vi "WPI_InterruptOpen.vi"(8 "error in (no error)":errorcluster, 9 "Falling Edge":bool, 10 "Rising Edge":bool, 11 "Source":T1={"DevStatus"={"status"=FALSE, "code"=0, "source"=""}, "AnalogTriggerMode?"=FALSE, "DigitalMode"={"DIO Channel"=enum."Disabled"}, "AnalogTriggerMode"={"AnalogTriggerIndex"=enum."Trig 0", "OutputType"=enum."InWindow"}}) -> (0 "error out":errorcluster, 3 "InterruptRef":T5={"DevStatus"={"status"=FALSE, "code"=0, "source"=""}, "InterruptIndex"=enum."Invalid"})   [LabVIEW 2017]
doc: "Opens a reference to the interrupt you specify. You must open a reference before using any other VIs on this palette.\n\nThis software is licensed. Open the labview\\readme\\WPI Robotics Library Open Source License.txt file for more information."
uses:
  <vilib>/Rock Robotics/WPI/Interrupt/WPI_InterruptRef.ctl
  <vilib>/Rock Robotics/SystemInterfaces/Interrupt/FPGA_InterruptIndex.ctl
  <vilib>/Rock Robotics/SystemInterfaces/CounterEncoderSourceConvertion/FPGA_CounterEncoderSourceConvertionLVSourceType.ctl
  <vilib>/Rock Robotics/SystemInterfaces/DIO/FPGA_DIODigitalSourceChannel.ctl
  <vilib>/Rock Robotics/SystemInterfaces/AnalogTrigger/FPGA_AnalogTriggerIndex.ctl
  <vilib>/Rock Robotics/SystemInterfaces/AnalogTrigger/FPGA_AnalogTriggerOutType.ctl
  <vilib>/Rock Robotics/WPI/Interrupt/WPI_InterruptCacheOp.ctl
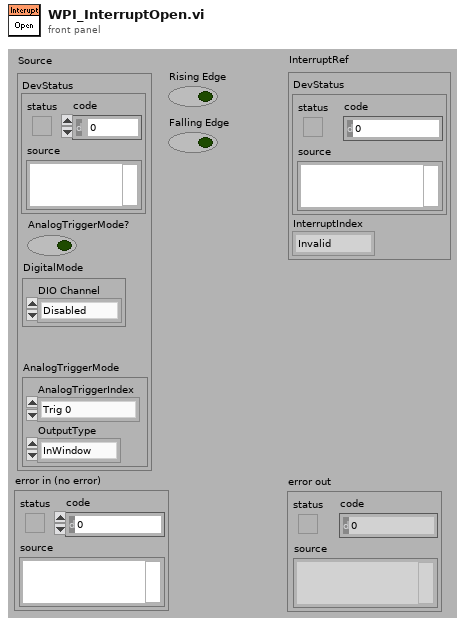
[diagram p1: front panel]
types:
  T1 = typedef "FPGA_CounterEncoderSourceConvertionLVSourceType.ctl" = cluster{"DevStatus":errorcluster, "AnalogTriggerMode?":bool, "DigitalMode":cluster{"DIO Channel":T2}, "AnalogTriggerMode":cluster{"AnalogTriggerIndex":T3, "OutputType":T4}}
  T2 = typedef "FPGA_DIODigitalSourceChannel.ctl" = enum8{"DIO 0", "DIO 1", "DIO 2", "DIO 3", "DIO 4", "DIO 5", "DIO 6", "DIO 7", "DIO 8", "DIO 9", "DIO MXP 0", "DIO MXP 1", "DIO MXP 2", "DIO MXP 3", "DIO MXP 4", "DIO MXP 5", "DIO MXP 6", "DIO MXP 7", "DIO MXP 8", "DIO MXP 9", "DIO MXP 10", "DIO MXP 11", "DIO MXP 12", "DIO MXP 13", "DIO MXP 14", "DIO MXP 15", "Disabled"}
  T3 = typedef "FPGA_AnalogTriggerIndex.ctl" = enum8{"Trig 0", "Trig 1", "Trig 2", "Trig 3", "Trig 4", "Trig 5", "Trig 6", "Trig 7", "Invalid"}
  T4 = typedef "FPGA_AnalogTriggerOutType.ctl" = enum16{"InWindow", "TriggerState", "Rising", "Falling"}
  T5 = typedef "WPI_InterruptRef.ctl" = cluster{"DevStatus":errorcluster, "InterruptIndex":T6}
  T6 = typedef "FPGA_InterruptIndex.ctl" = enum8{"0", "1", "2", "3", "4", "5", "6", "7", "Invalid"}
  T7 = typedef "WPI_InterruptCacheOp.ctl" = enum16{"Acquire", "Release"}
  T8 = typedef "FPGA_InterruptRef.ctl" = cluster{"DevStatus":errorcluster, "Interrupt Index":T6}
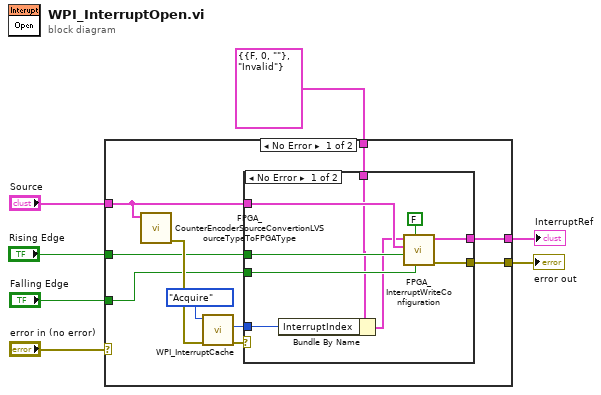
[diagram p0: block diagram]
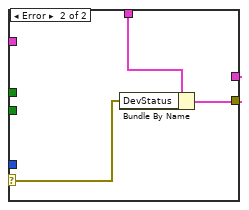
[diagram p2: hidden frame]
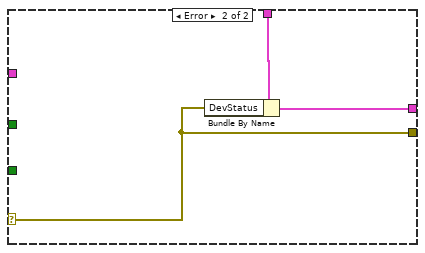
[diagram p3: hidden frame]
diagram:
  n1 = case shown="No Error" "error in (no error)" {
    selector: "error in (no error)" -> [_ w30]
    tunnel: [w17 w31] -> w4
    tunnel: T5 {"DevStatus"={"status"=FALSE, "code"=0, "source"=""}, "InterruptIndex"=enum."Invalid"} ("InteruptRef") -> [w16 w32]
    tunnel: [w15 w30] -> w6
    tunnel: "Source" -> [w12 _]
    tunnel: "Rising Edge" -> [w9 _]
    tunnel: "Falling Edge" -> [w8 _]
    frame No Error {
      n2 = call <vilib>:"FPGA_CounterEncoderSourceConvertionLVSourceTypeToFPGAType.vi"("DigitalSource"=w12) -> ("error out"=w11:errorcluster)  [unwired: 1 in, 9 out]
      n3 = call <vilib>:"WPI_InterruptCache.vi"("error in (no error)"=w11, "InterruptCacheOp"=WPI_InterruptCacheOp."Acquire" ("InteruptCacheOp")) -> ("error out"=w14:errorcluster, "InterruptIndexAllocated"=w13:T6)  [unwired: 8 out]
      n4 = case shown="No Error" w14 {
        selector: w14 -> [_ w27]
        tunnel: [w19 w28] -> w17
        tunnel: w16 -> [w21 w29]
        tunnel: [w26 w27] -> w15
        tunnel: w13 -> [w22 _]
        tunnel: w12 -> [w25 _]
        tunnel: w9 -> [w24 _]
        tunnel: w8 -> [w23 _]
        frame No Error {
          n5 = Bundle By Name(cluster=w21, "InterruptIndex"=w22) -> (w20:T5)
          n6 = call <vilib>:"FPGA_InterruptWriteConfiguration.vi"("Falling Edge"=w23, "WaitForAck"=FALSE, "Rising Edge"=w24, "Source"=w25, "InteruptRef in"=w20) -> ("error out"=w26:errorcluster, "InteruptRef out"=w19:T8)  [unwired: 1 in, 4 out]
        }
        frame Error {
          n7 = Bundle By Name(cluster=w29, "DevStatus"=w27) -> (w28:T5)
        }
      }
    }
    frame Error {
      n8 = Bundle By Name(cluster=w32, "DevStatus"=w30) -> (w31:T5)
    }
  }
  "InterruptRef" <- w4
  "error out" <- w6
